vi "LOER_SelectMenu.vi"(0 "XRef":T11, 1 "Tag":T6, 2 "Point":T9, 3 "Menu Type":T8, 4 "State In":T1={"Inputs"=1, "SelectedIndex"=0, "ClassInfo"=[], "Width"=100, "EventReg Type"=variant}) -> (14 "Reply":T5, 15 "Handled?":T7, 16 "Multi Object Popup Options":T4, 17 "Fatal Error Out":T3, 18 "State Out":T1={"Inputs"=1, "SelectedIndex"=0, "ClassInfo"=[], "Width"=100, "EventReg Type"=variant})   [LabVIEW 2016, in "LV Object Event Registration Node.xnode"]
uses:
  LV Object Event Registration Node.xnode
  <vilib>/XNodeSupport/XNodeXNodeRef.ctl
  <vilib>/XNodeSupport/XNodeString.ctl
  <vilib>/XNodeSupport/XNodePoint.ctl
  <vilib>/XNodeSupport/XNodeInt.ctl
  <vilib>/XNodeSupport/XNodeMenuType.ctl
  LOER_State.ctl
  LOER_ClassInfo.ctl
  <vilib>/XNodeSupport/XNodeStringArray.ctl
  <vilib>/XNodeSupport/XNodeBool.ctl
  <vilib>/XNodeSupport/XNodeMultiObjectPopupOptions.ctl
  <vilib>/XNodeSupport/XNodeErrorCluster.ctl
  <vilib>/XNodeSupport/NI_XNodeSupport.lvlib
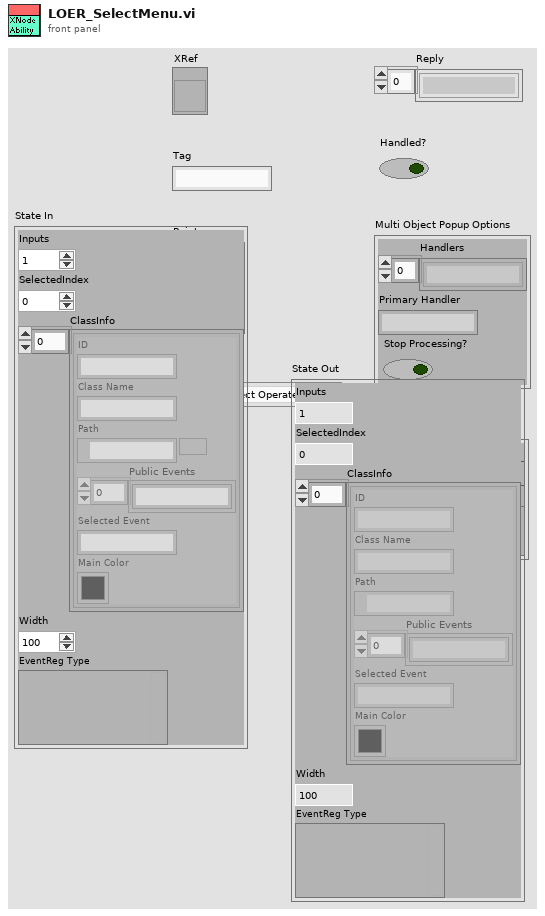
[diagram p1: front panel]
types:
  T1 = typedef "LV Object Event Registration Node.xnode/LOER_State.ctl" = cluster{"Inputs":u16, "SelectedIndex":i16, "ClassInfo":T2[], "Width":u16, "EventReg Type":variant}
  T2 = typedef "LV Object Event Registration Node.xnode/LOER_ClassInfo.ctl" = cluster{"ID":string, "Class Name":string, "Path":path, "Public Events":string[], "Selected Event":string, "Main Color":u32}
  T3 = typedef "NI_XNodeSupport.lvlib/XNodeErrorCluster.ctl" = errorcluster
  T4 = typedef "NI_XNodeSupport.lvlib/XNodeMultiObjectPopupOptions.ctl" = cluster{"Handlers":T5, "Primary Handler":T6, "Stop Processing?":T7}
  T5 = typedef "NI_XNodeSupport.lvlib/XNodeStringArray.ctl" = T6[]
  T6 = typedef "NI_XNodeSupport.lvlib/XNodeString.ctl" = string
  T7 = typedef "NI_XNodeSupport.lvlib/XNodeBool.ctl" = bool
  T8 = typedef "NI_XNodeSupport.lvlib/XNodeMenuType.ctl" = enum32{"Single Object Operate", "Single Object Popup", "Multi Object Popup Master", "Multi Object Popup Other"}
  T9 = typedef "NI_XNodeSupport.lvlib/XNodePoint.ctl" = cluster{"H":T10, "V":T10}
  T10 = typedef "NI_XNodeSupport.lvlib/XNodeInt.ctl" = i32
  T11 = typedef "NI_XNodeSupport.lvlib/XNodeXNodeRef.ctl" = refnum<vi>
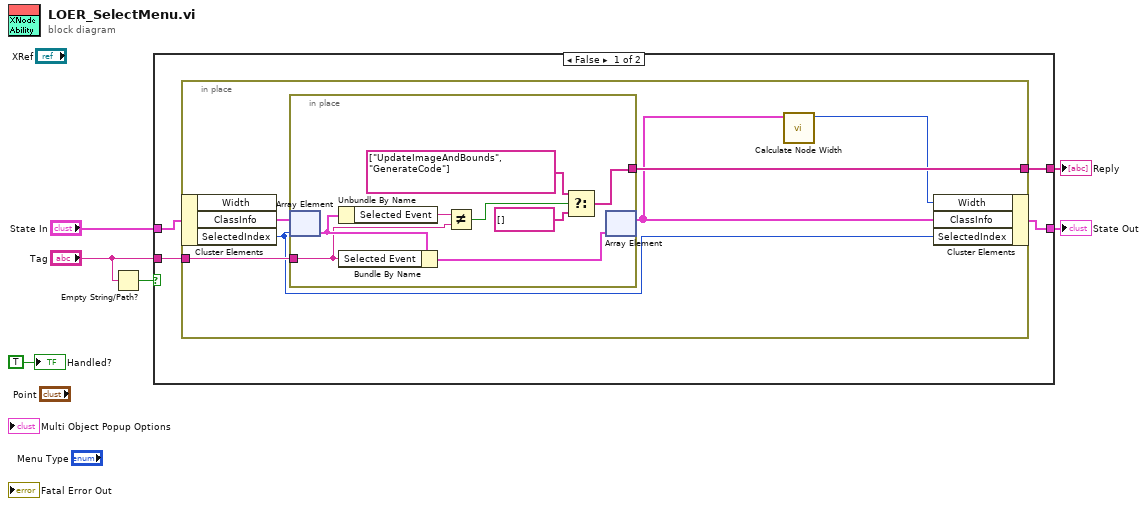
[diagram p0: block diagram]
diagram:
  n1 = Empty String/Path?(string/path="Tag") -> (empty?=w2:bool)
  n2 = case shown="False" w2 {
    tunnel: "Tag" -> [w10 _]
    tunnel: "State In" -> [w9 w25]
    tunnel: [w8 w25] -> w5
    tunnel: [w7 _] -> w3
    frame False {
      n3 = in-place {
        in-place-border: w10 -> [w16]
        in-place-border: [w14] -> w7
        n4 = in-place-cluster #1(w9) -> ("ClassInfo"=w15:T2[], "SelectedIndex"=w13:i16)  [unwired: 1 out]
        n5 = in-place {
          in-place-border: w16 -> [w17]
          in-place-border: [w18] -> w14
          n6 = in-place-array #2(w15, w13) -> (w23:T2)
          n7 = Unbundle By Name(w23) -> ("Selected Event"=w22:string)
          n8 = Bundle By Name(cluster=w23, "Selected Event"=w17) -> (w24:T2)
          n9 = Not Equal?(x=w22, y=w17) -> (x != y?=w21:bool)
          n10 = Select(t=T5 ["UpdateImageAndBounds", "GenerateCode"] ("Reply"), s=w21, f=T5 [] ("Reply")) -> (s? t:f=w18:T5)
          n11 = in-place-array #2(w24) -> (w12:T2[])  [unwired: 1 out]
        }
        n12 = call "Calculate Node Width.vi"("ClassInfo"=w12) -> ("upper limit"=w11:i16)  [unwired: 10 in]
        n13 = in-place-cluster #1("Width"=w11, "ClassInfo"=w12, "SelectedIndex"=w13) -> (w8:T1)
      }
    }
    frame True {
    }
  }
  "Reply" <- w3
  "State Out" <- w5
  "Handled?" <- T7 TRUE ("Handled?")
